vi "Read.vi"(8 "error in (no error)":errorcluster, 11 "Reference in":T1={"Device"="GPIB0::4::INSTR", "Function"="", "delay"=20}) -> (0 "error out":errorcluster, 1 "value":dbl, 3 "Reference out":T1={"Device"="GPIB0::4::INSTR", "Function"="", "delay"=20}, 4 "question out":string)   [LabVIEW 2021, in "Rigol DM3052.lvlib"]
uses:
  Rigol DM3052.lvlib
  Reference.ctl
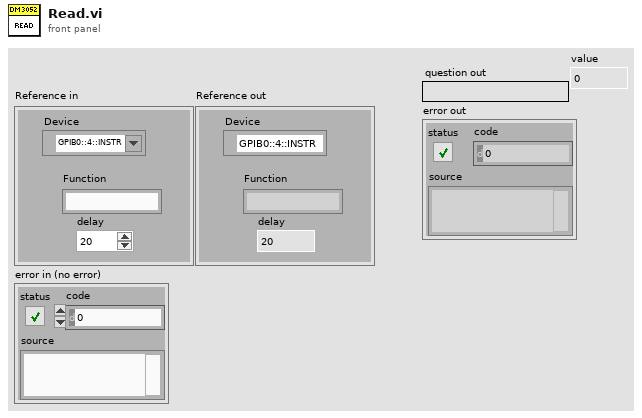
[diagram p1: front panel]
types:
  T1 = typedef "Rigol DM3052.lvlib/Reference.ctl" = cluster{"Device":refnum<visa-resource-name>, "Function":string, "delay":u32}
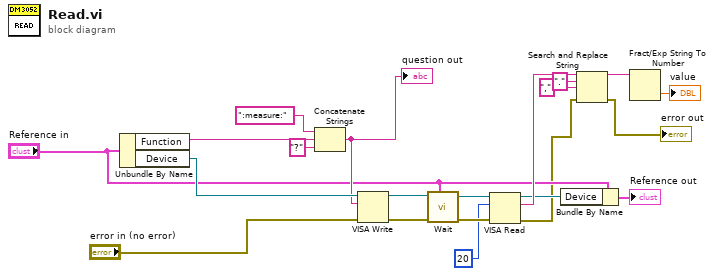
[diagram p0: block diagram]
diagram:
  n1 = Unbundle By Name("Reference in") -> ("Function"=w19:string, "Device"=w21:refnum<visa-resource-name>)
  n2 = Concatenate Strings(":measure:" ("string"), w19, "?" ("string")) -> (w12:string)
  "question out" <- w12
  n3 = VISA Write(VISA resource name=w21, write buffer=w12, error in (no error)="error in (no error)") -> (VISA resource name out=w16:refnum<visa-resource-name>, error out=w15:errorcluster)  [unwired: 1 out]
  n4 = call "Wait.vi"("Reference in"="Reference in", "error in (no error)"=w15, "Device in"=w16) -> ("error out"=w13:errorcluster, "Device out"=w14:refnum<visa-resource-name>)  [unwired: 7 in]
  n5 = VISA Read(VISA resource name=w14, byte count=u32 20, error in (no error)=w13) -> (VISA resource name out=w9:refnum<visa-resource-name>, read buffer=w11:string, error out=w4:errorcluster)  [unwired: 1 out]
  n6 = Bundle By Name(cluster="Reference in", "Device"=w9) -> (→"Reference out":T1)
  n7 = Search and Replace String(input string=w11, search string=".", replace string="," ("replace string (\"\")"), error in=w4) -> (result string=w5:string, error out=→"error out":errorcluster)  [unwired: 4 in, 2 out]
  n8 = Fract/Exp String To Number(string=w5) -> (number=→"value":dbl)  [unwired: 3 in, 1 out]
